vi "Countdown.vi"(7 "reset":bool, 11 "countdownFrom":i32) -> (0 "finished":bool, 3 "counter":i32)   [LabVIEW 2010, in "kevLib2011.lvlib"]
uses:
  kevLib2011.lvlib
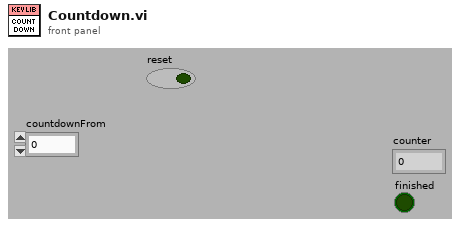
[diagram p1: front panel]
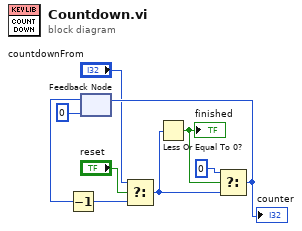
[diagram p0: block diagram]
diagram:
  n1 = feedback #1(0) -> (w9:i32)
  n2 = Decrement(x=w9) -> (x-1=w3:i32)
  n3 = Select(t="countdownFrom", s="reset", f=w3) -> (s? t:f=w1:i32)
  n4 = Less Or Equal To 0?(x=w1) -> (x <= 0?=w8:bool)
  "finished" <- w8
  n5 = Select(t=0, s=w8, f=w1) -> (s? t:f=w6:i32)
  "counter" <- w6
  n6 = feedback-in #1(w6) -> ()
